vi "OpenByPath.vi"(0 "VI path":path, 1 "Application reference":refnum<vi> caption="Application reference (Local)", 9 "Reentrancy mode":T2=enum."Auto" caption="Reentrancy mode (Auto)", 11 "Error in":errorcluster caption="Error in (no error)") -> (4 "VI refnum out":refnum<vi>, 6 "VI refnum opened?":bool, 8 "Last execution state":T1(ring), 10 "VI refnum opened as reentrant?":bool, 15 "Error out":errorcluster)   [LabVIEW 2017, in "VILauncher.lvlib"]
doc: "Opens a reference to a dynamic VI specified by <B>VI path</B> and returns the reference to the opened VI in <B>VI refnum out</B>. Remember to close the VI reference when you're done using it.\n\nThe optional <B>Application reference</B> can be used to specify another application instance to open the VI reference in. Use the Open Application Reference LabVIEW function to open another application reference.\n\nUse the optional <B>Reentrancy mode</B> input to specify whether the dynamic VI should be opened as a reentrant or a non-reentrant instance. Set this to Auto (default) to first try as reentrant, and if that fails, as non-reentrant. The <B>VI refnum opened as reentrant?</B> output will reflect the instantiation mode.\n\nThe <B>VI refnum opened?</B> output will only be True if the dynamic VI's <B>Last execution state</B> is \"Idle\" or \"Running\".\n\nThis VI is reentrant, and it doesn't run if there is an error on <B>Error in</B>.\n\nSteen Schmidt\nGPower\n26/12 2012"
uses:
  VILauncher.lvlib
  Error/GPError.lvlib
  Typedefs/ReentrancyMode.ctl
panel:
  # "Copyright © 2013\nGPower\nSee enclosed license file for terms and conditions"
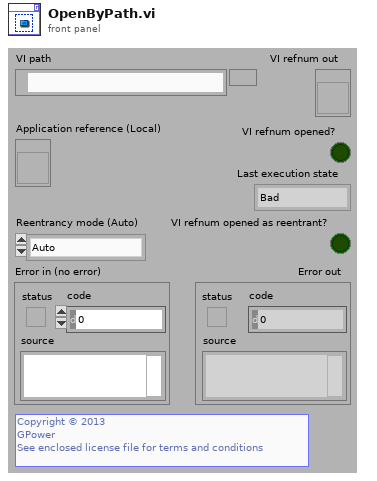
[diagram p1: front panel]
types:
  T1 = enum32{"Bad", "Idle", "Run top level", "Running"}
  T2 = typedef "VILauncher.lvlib/ReentrancyMode.ctl" = enum16{"Reentrant", "Non-reentrant", "Auto"}
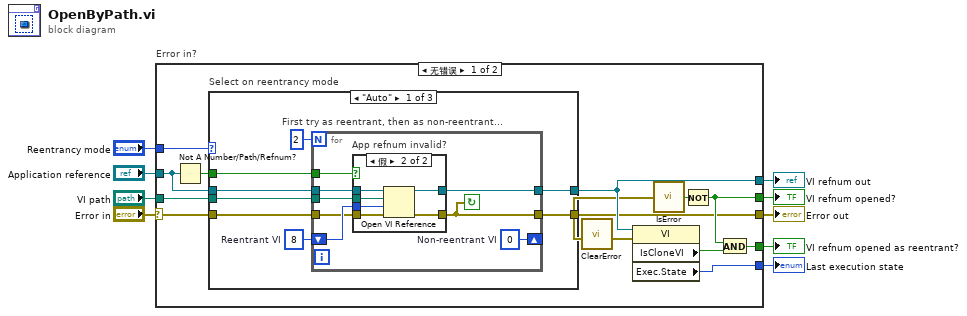
[diagram p0: block diagram]
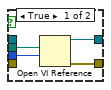
[diagram p2: hidden frame]
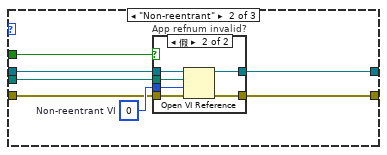
[diagram p3: hidden frame]
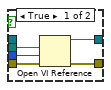
[diagram p4: hidden frame]
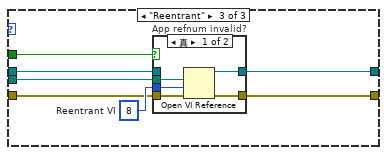
[diagram p5: hidden frame]
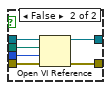
[diagram p6: hidden frame]
diagram:
  n1 = case "Error in?" shown="无错误" "Error in" {
    selector: "Error in" -> [w15 w85]
    tunnel: [w10 w85] -> w8
    tunnel: "VI path" -> [w22 _]
    tunnel: "Application reference" -> [w17 _]
    tunnel: "Reentrancy mode" -> [w20 _]
    tunnel: [w12 _] -> w4
    tunnel: [w19 _] -> w3
    tunnel: [w13 _] -> w2
    tunnel: [w18 _] -> w1
    frame No Error {
      n2 = Not A Number/Path/Refnum?(number/path/refnum=w17) -> (NaN/Path/Refnum?=w16:bool)
      n3 = case "Select on reentrancy mode" shown="\"Auto\"" w20 {
        tunnel: w22 -> [w28 w51 w69]
        tunnel: w17 -> [w27 w52 w70]
        tunnel: [w26 w54 w72] -> w18
        tunnel: [w25 w55 w73] -> w10
        tunnel: w16 -> [w24 w53 w71]
        tunnel: w15 -> [w23 w49 w67]
        frame "Auto" {
          w30 = 8  # Reentrant VI
          n4 = for "First try as reentrant, then as non-reentrant..." {
            N: 2 -> [_]
            shift-right: [w37] -> _
            shift-left: w30 -> [w38]
            tunnel: w28 -> [w36]
            tunnel: w27 -> [w35]
            tunnel: [w34] -> w26
            tunnel: [w33] -> w25
            tunnel: w24 -> [w32]
            tunnel: w23 -> [w31]
            stop <- w33 continue-if-true
            w37 = 0  # Non-reentrant VI
            n5 = case "App refnum invalid?" shown="假" w32 {
              tunnel: w38 -> [w42 w48]
              tunnel: w36 -> [w41 w47]
              tunnel: w35 -> [_ w46]
              tunnel: [w40 w45] -> w34
              tunnel: [w39 w44] -> w33
              tunnel: w31 -> [_ w43]
              frame True {
                n6 = Open VI Reference(vi path=w41, options=w42) -> (vi reference=w40:refnum<vi>, error out=w39:errorcluster)  [unwired: 2 in, 2 out]
              }
              frame False {
                n7 = Open VI Reference(application reference (local)=w46, vi path=w47, options=w48, error in (no error)=w43) -> (vi reference=w45:refnum<vi>, error out=w44:errorcluster)  [unwired: 1 in, 1 out]
              }
            }
          }
        }
        frame "Non-reentrant" {
          w50 = 0  # Non-reentrant VI
          n8 = case "App refnum invalid?" shown="假" w53 {
            tunnel: w50 -> [w60 w66]
            tunnel: w51 -> [w59 w65]
            tunnel: w52 -> [_ w64]
            tunnel: [w58 w63] -> w54
            tunnel: [w57 w62] -> w55
            tunnel: w49 -> [w56 w61]
            frame True {
              n9 = Open VI Reference(vi path=w59, options=w60, error in (no error)=w56) -> (vi reference=w58:refnum<vi>, error out=w57:errorcluster)  [unwired: 1 in, 2 out]
            }
            frame False {
              n10 = Open VI Reference(application reference (local)=w64, vi path=w65, options=w66, error in (no error)=w61) -> (vi reference=w63:refnum<vi>, error out=w62:errorcluster)  [unwired: 1 in, 1 out]
            }
          }
        }
        frame "Reentrant" {
          w68 = 8  # Reentrant VI
          n11 = case "App refnum invalid?" shown="真" w71 {
            tunnel: w68 -> [w78 w84]
            tunnel: w69 -> [w77 w83]
            tunnel: w70 -> [_ w82]
            tunnel: [w76 w81] -> w72
            tunnel: [w75 w80] -> w73
            tunnel: w67 -> [w74 w79]
            frame True {
              n12 = Open VI Reference(vi path=w77, options=w78, error in (no error)=w74) -> (vi reference=w76:refnum<vi>, error out=w75:errorcluster)  [unwired: 1 in, 2 out]
            }
            frame False {
              n13 = Open VI Reference(application reference (local)=w82, vi path=w83, options=w84, error in (no error)=w79) -> (vi reference=w81:refnum<vi>, error out=w80:errorcluster)  [unwired: 1 in, 1 out]
            }
          }
        }
      }
      n14 = call "ClearError.vi"("Error in"=w10) -> ("Error out"=w21:errorcluster)  [unwired: 10 in]
      n15 = property class="VI"(reference=w18, error in=w21) -> ("IsCloneVI"=w11:bool, "Exec.State"=w13:T1)  [unwired: 2 out]
      n16 = call "IsError.vi"("Error in"=w10) -> ("Error?"=w14:bool)  [unwired: 4 in]
      n17 = Not(x=w14) -> (.not. x?=w12:bool)
      n18 = And(x=w12, y=w11) -> (x .and. y?=w19:bool)
    }
    frame Error {
    }
  }
  "Error out" <- w8
  "VI refnum out" <- w1
  "Last execution state" <- w2
  "VI refnum opened as reentrant?" <- w3
  "VI refnum opened?" <- w4
